vi "ErrorHandling.Create.vi"(6 "skip levels (0)":i32, 7 "error code (5000)":i32(ring)=5000 items=["No error", "Argument error", "Memory is full", "Out of zone", "End of file", "File already open", "Generic file I/O error", "File not found", "File permission error", "Disk is full", "Duplicate path", "Too many files open", "System feature not enabled", "Resource file not found", "Cannot add resource", "Resource not found", "Image not found", "Image memory error", "Pen does not exist", "Config type invalid", "Config token not found", "Config parse error", "Config memory error", "Bad external code format", "Bad external code offset", "External code not present", "Null window", "Destroy window error", "Null menu", "Print aborted", "Bad print record", "Print driver error", "Windows error during printing", "Memory error during printing", "Print dialog error", "Generic print error", "Invalid device refnum", "Device not found", "Device parameter error", "Device unit error", "Cannot open device", "Device call aborted", "Generic error", "Cancelled by user", "Object ID too low", "Object ID too high", "Object not in heap", "Unknown heap", "Unknown object (invalid DefProc)", "Unknown object (DefProc not in table)", "Message out of range", "Invalid (null) method", "Unknown message", "Manager call not supported", "Bad address", "Network operation in progress", "Network operation timed out", "Connection is busy", "Network attribute not supported", "Network error", "Address in use", "System out of memory", "Connection aborted", "Connection refused", "Not connected", "Already connected", "Connection closed", "Initialization error (interapplication manager)", "Bad occurrence", "Wait on unbound occurrence handler", "Occurrence queue overflow", "Datalog type conflict", "Unused", "Unrecognized type (interapplication manager)", "Memory corrupt", "Failed to make temporary DLL", "Old CIN version", "Drag socket not found", "Failed to load drop-object", "Failed to register OLE object", "Failed to release OLE object", "Format specifier type mismatch", "Unknown format specifier", "Too few format specifiers", "Too many format specifiers", "Scan failed", "Newer CIN version", "Error converting to variant", "Runtime menu error", "Password tampered", "Variant attribute not found", "Incompatible variant data type", "Event data is not available", "Event Store is not present", "Occurrence is not found", "Event Queue is not created", "Event info is not available", "Refnum passed is NULL", "Error retrieving Class GUID", "Error retrieving CoClass GUID", "Error retrieving TypeLib GUID.", "Bad built application magic bytes.", "Specific driver is different from the specific driver associated with the Logical Name.", "There is no session opened to the class driver.", "Max Error", "MAX - Error with config objects", "MAX - Error loading configuration", "MAX - Group not supported"], 8 "error in":errorcluster, 9 "warning only (F)":bool, 10 "explanation":string, 11 "create (T)":bool=TRUE) -> (0 "error out":errorcluster)   [LabVIEW 2019, in "Tools.lvlib"]
doc: "Creates an error in the error wire.\nIf an error is present in <B>error in</B>, it will be passed on without any further action.\n\nOnly actually creates the error if <B>create</B>=True (default).\nIn the text of the error the source VI and call trace is added, as well as the time.\n\nA message that you could attach to the <B>explanation</B> input could be the following lines:\n Invalid config file format.\n File: C:\\myapp\\savetheworld.ini"
uses:
  Tools.lvlib
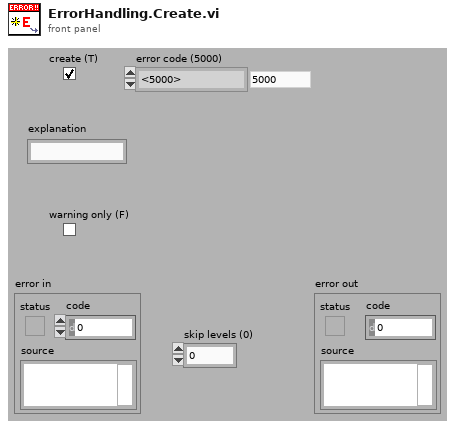
[diagram p1: front panel]
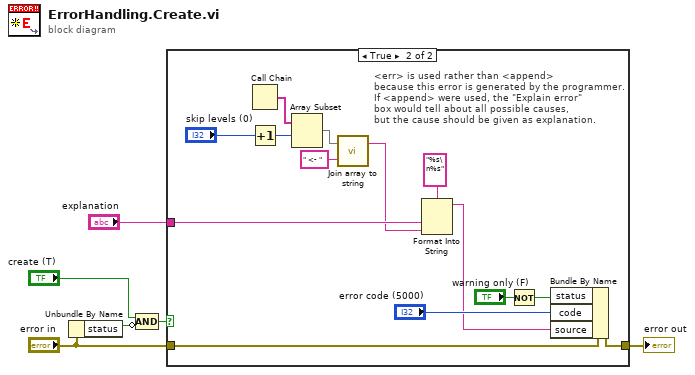
[diagram p0: block diagram]
diagram:
  n1 = Unbundle By Name("error in") -> ("status"=w5:bool)
  n2 = Compound Arithmetic op=AND("create (T)", invert w5) -> (w3:bool)
  n3 = case shown="True" w3 {
    tunnel: [w7 w21] -> w6
    tunnel: "error in" -> [w7 w15]
    tunnel: "explanation" -> [_ w9]
    frame False {
    }
    frame True {
      # "<err> is used rather than <append>\nbecause this error is generated by the programmer.\nIf <append> were used, the \"Explain error\"\nbox would tell about all possible causes,\nbut the cause should be given as explanation."
      n4 = Call Chain() -> (call chain=w18:string[])
      n5 = Increment(x="skip levels (0)") -> (x+1=w16:i32)
      n6 = Array Subset(array=w18, index=w16) -> (w17:string[])  [unwired: 1 in]
      n7 = call "Join array to string.vi"("Delimiter (,)"=" <- ", "String array"=w17) -> ("Joined elements"=w8:string)  [unwired: 1 out]
      n8 = Format Into String(format string="%s\n%s" ("string"), w9, w8) -> (resulting string=w11:string)  [unwired: 2 in, 1 out]
      n9 = Not(x="warning only (F)") -> (.not. x?=w14:bool)
      n10 = Bundle By Name(cluster=w15, "status"=w14, "code"="error code (5000)", "source"=w11) -> (w21:errorcluster)
    }
  }
  "error out" <- w6
